vi "Unflatten Value.vi"(8 "error in (no error)":errorcluster, 10 "Value":string, 11 "Boolean in":refnum<class "U32.lvclass">) -> (0 "error out":errorcluster, 3 "Boolean out":refnum<class "U32.lvclass">)   [LabVIEW 2020, in "U32.lvclass"]
uses:
  <vilib>/gpm_packages/@cs/data-type-serializer/source/U32/U32.lvclass
  <vilib>/gpm_packages/@cs/data-type-serializer/source/U32/U32.lvclass/U32.ctl
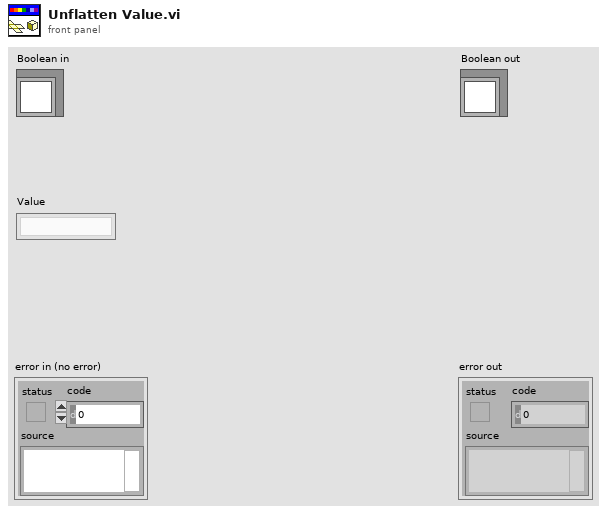
[diagram p1: front panel]
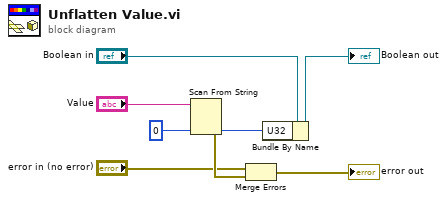
[diagram p0: block diagram]
diagram:
  n1 = Scan From String(input string="Value", default 1=u32 0) -> (error out=w6:errorcluster, output 1=w5:u32)  [unwired: 3 in, 2 out]
  n2 = Merge Errors("error in (no error)", w6) -> (→"error out":errorcluster)
  n3 = Bundle By Name(cluster="Boolean in", "U32"=w5) -> (→"Boolean out":refnum<class "U32.lvclass">)
